vi "Stop Core.vi"(10 "final error code":i32, 11 "Actor ErrorStop in":refnum<class "Actor ErrorStop.lvclass">) -> (3 "Actor ErrorStop out":refnum<class "Actor ErrorStop.lvclass">)   [LabVIEW 2012, in "Actor ErrorStop.lvlib" / "Actor ErrorStop.lvclass"]
doc: "(<B>Filename</B>: Actor Framework.lvlib:Actor.lvclass:Stop Core.vi)\n\nDefines what the actor does before it stops. Use the <B>final error code</B> input to determine whether the actor shut down in response to an error.\n\nBy default, this method does nothing. A descendant class may override it to define behavior, such as shutting down any processes the actor initiated in its override of the Actor Core method."
uses:
  Actor ErrorStop.lvclass
  <vilib>/ActorFramework/Actor/Actor.lvclass
  Actor ErrorStop.lvclass/Actor ErrorStop.ctl
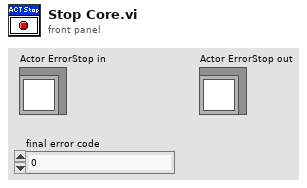
[diagram p1: front panel]
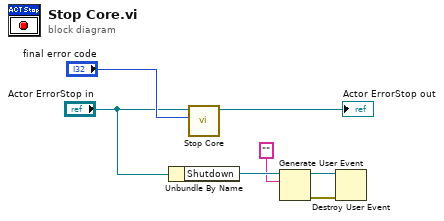
[diagram p0: block diagram]
diagram:
  n1 = Unbundle By Name("Actor ErrorStop in") -> ("Shutdown"=w4:refnum<user-event>)
  n2 = call-parent "Stop Core.vi"("final error code"="final error code", "Actor in"="Actor ErrorStop in") -> ("Actor out"=→"Actor ErrorStop out":refnum<class "Actor ErrorStop.lvclass">)  [unwired: 9 in]
  n3 = Generate User Event(user event=w4, event data cluster="" ("event data")) -> (user event out=w2:refnum<user-event>, error out=w1:errorcluster)  [unwired: 1 in]
  n4 = Destroy User Event(user event=w2, error in=w1) -> ()  [unwired: 1 out]
